vi "BeepServer.vi"(8 "error in":errorcluster) -> (0 "error out":errorcluster)   [LabVIEW 2010, in "Labricks.lvlib" / "Game.lvclass"]
uses:
  Game.lvclass
  <vilib>/sound2/lvsound2.llb/Sound Data Format.ctl
  <vilib>/sound2/lvsound2.llb/Sampling Mode.ctl
  <vilib>/sound2/lvsound2.llb/Sound Output Write (DBL Single).vi
  <vilib>/measure/NI_MABase.lvlib
panel:
  in  "device ID":u32
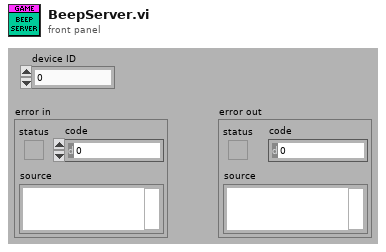
[diagram p1: front panel]
types:
  T1 = typedef "Sampling Mode.ctl" = i32
  T2 = typedef "Sound Data Format.ctl" = cluster{"sample rate (S/s)":dbl, "number of channels":i32, "bits per sample":i32}
  T3 = typedef "Sound Output Task ID.ctl" = u32
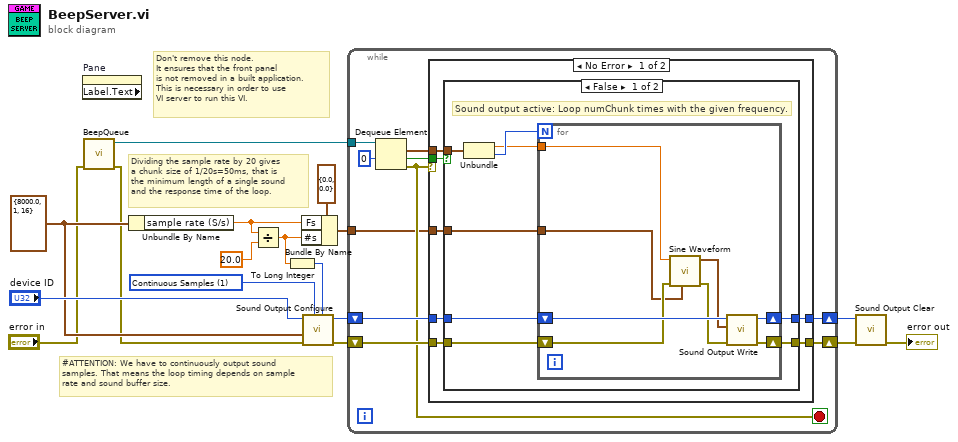
[diagram p0: block diagram]
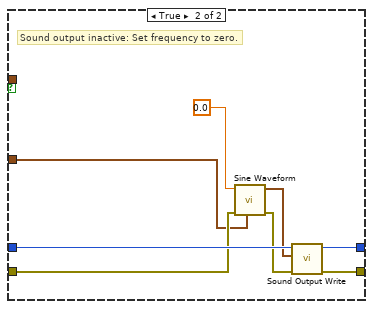
[diagram p2: hidden frame]
diagram:
  w11 = T1 1 items=["Finite Samples", "Continuous Samples"] ("sample mode")
  w10 = T2 {"sample rate (S/s)"=8000.0, "number of channels"=1, "bits per sample"=16} ("sound format")
  # "Don't remove this node.\nIt ensures that the front panel\nis not removed in a built application.\nThis is necessary in order to use\nVI server to run this VI."
  # "#ATTENTION: We have to continuously output sound\nsamples. That means the loop timing depends on sample\nrate and sound buffer size."
  # "Dividing the sample rate by 20 gives\na chunk size of 1/20s=50ms, that is\nthe minimum length of a single sound\nand the response time of the loop."
  n1 = property on="Pane" class="Pane" props=["Label", "Text"]() -> ()  [unwired: 2 in, 3 out]
  n2 = call "BeepQueue.vi"("error in"="error in") -> ("error out"=w6:errorcluster, "queue out"=w7:refnum<queue>)  [unwired: 5 in]
  n3 = Unbundle By Name(w10) -> ("sample rate (S/s)"=w2:dbl)
  n4 = Divide(x=w2, y=20.0) -> (x/y=w4:dbl)
  n5 = To Long Integer(number=w4) -> (32bit integer=w8:i32)
  n6 = Bundle By Name(cluster=cluster{"Fs":dbl, "#s":dbl} {"Fs"=0.0, "#s"=0.0} ("sampling info"), "Fs"=w2, "#s"=w4) -> (w1:cluster{"Fs":dbl, "#s":dbl})
  n7 = call <vilib>:"Sound Output Configure.vi"("number of samples/ch"=w8, "sample mode"=w11, "error in (no error)"=w6, "sound format"=w10, "device ID"="device ID") -> ("error out"=w12:errorcluster, "task ID"=w13:T3)  [unwired: 2 in, 3 out]
  n8 = while {
    shift-right: [w27] -> w16
    shift-left: w13 -> [w26]
    shift-right: [w24] -> w17
    shift-left: w12 -> [w23]
    tunnel: w7 -> [w25]
    tunnel: w1 -> [w18]
    stop <- w22 stop-if-true
    n9 = Dequeue Element(queue=w25, timeout in ms (-1)=0) -> (element=w20:cluster{"frequency":dbl, "duration":i32}, timed out?=w21:bool, error out=w22:errorcluster)  [unwired: 1 in, 1 out]
    n10 = case shown="No Error" w22 {
      tunnel: [w34 w60] -> w27
      tunnel: w26 -> [w33 w60]
      tunnel: w20 -> [w30 _]
      tunnel: [w32 w59] -> w24
      tunnel: w23 -> [w31 w59]
      tunnel: w21 -> [w29 _]
      tunnel: w18 -> [w28 _]
      frame No Error {
        n11 = case shown="False" w29 {
          tunnel: [w42 w58] -> w34
          tunnel: w33 -> [w41 w57]
          tunnel: [w40 w56] -> w32
          tunnel: w31 -> [w39 w55]
          tunnel: w30 -> [w38 _]
          tunnel: w28 -> [w36 w51]
          frame False {
            # "Sound output active: Loop numChunk times with the given frequency."
            n12 = Unbundle(w38) -> ("frequency"=w35:dbl, "duration"=w37:i32)
            n13 = for {
              N: w37 -> [_]
              shift-right: [w50] -> w42
              shift-left: w41 -> [w49]
              shift-right: [w48] -> w40
              shift-left: w39 -> [w47]
              tunnel: w36 -> [w44]
              tunnel: w35 -> [w43]
              n14 = call <vilib>:"Sine Waveform.vi"("sampling info"=w44, "error in (no error)"=w47, "frequency"=w43) -> ("error out"=w45:errorcluster, "signal out"=w46:waveform(dbl))  [unwired: 7 in]
              n15 = call-poly <vilib>:"Sound Output Write.vi"("error in (no error)"=w45, "data"=w46, "task ID"=w49) -> ("error out"=w48:errorcluster, "task ID out"=w50:T3)  [unwired: 1 in, 6 out]
            }
          }
          frame True {
            # "Sound output inactive: Set frequency to zero."
            n16 = call <vilib>:"Sine Waveform.vi"("sampling info"=w51, "error in (no error)"=w55, "frequency"=0.0) -> ("error out"=w53:errorcluster, "signal out"=w54:waveform(dbl))  [unwired: 7 in]
            n17 = call-poly <vilib>:"Sound Output Write.vi"("error in (no error)"=w53, "data"=w54, "task ID"=w57) -> ("error out"=w56:errorcluster, "task ID out"=w58:T3)  [unwired: 1 in, 6 out]
          }
        }
      }
      frame Error {
      }
    }
  }
  n18 = call <vilib>:"Sound Output Clear.vi"("error in (no error)"=w17, "task ID"=w16) -> ("error out"=→"error out":errorcluster)  [unwired: 9 out]
